vi "GetText.vi"(8 "error in":errorcluster, 11 "node in":refnum<class "RunTimeButton.lvclass">) -> (0 "error out":errorcluster, 1 "additional text":string, 2 "text":string, 3 "node out":refnum<class "RunTimeButton.lvclass">, 4 "glyph":string)   [LabVIEW 2015, in "RunTimeButton.lvclass"]
doc: "Returns the text representation of the node used for the tree control."
uses:
  RunTimeButton.lvclass
  RunTimeButton.lvclass/RunTimeButton.ctl
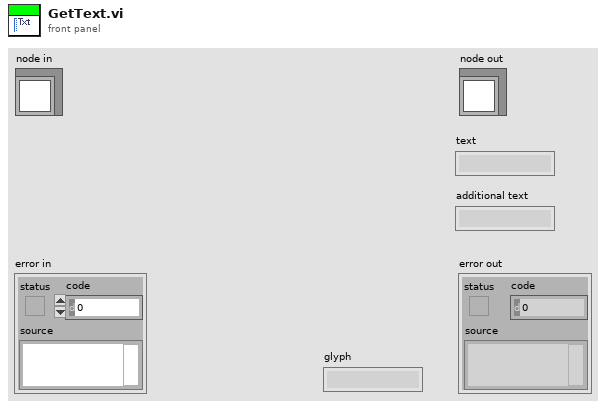
[diagram p1: front panel]
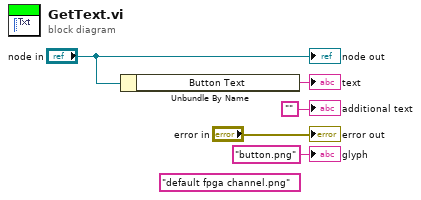
[diagram p0: block diagram]
diagram:
  (unwired) "default fpga channel.png" ("glyph")
  n1 = Unbundle By Name("node in") -> ("Button Text"=→"text":string)
  "error out" <- "error in"
  "node out" <- "node in"
  "additional text" <- ""
  "glyph" <- "button.png" ("glyph")
